vi "Package Class FG.vi"(8 "error in (no error)":errorcluster, 10 "Package Type (All)":string) -> (0 "error out":errorcluster, 2 "Package Class":refnum<class "PackageAbstract.lvclass">, 3 "Package Classes":T1(c390))   [LabVIEW 2020, in "GPack.lvlib"]
uses:
  GPack.lvlib
  PackageAbstract/PackageAbstract.lvclass
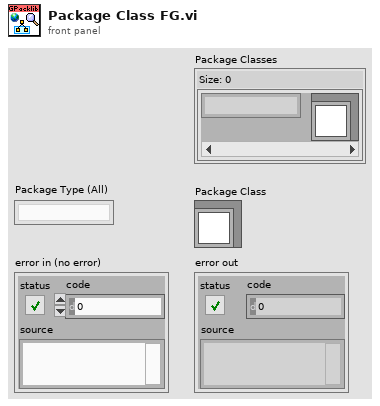
[diagram p1: front panel]
types:
  T1 = map{string, refnum<class "PackageAbstract.lvclass">}
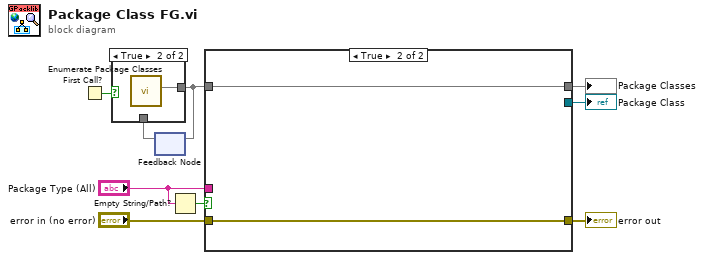
[diagram p0: block diagram]
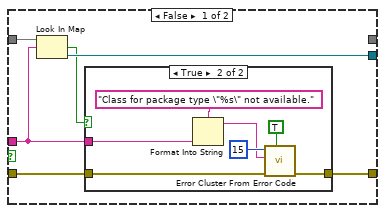
[diagram p3: hidden frame]
diagram:
  n1 = First Call?() -> (First Call?: T/F=w9:bool)
  n2 = feedback #1() -> (w8:T1)  [unwired: 1 in]
  n3 = case shown="True" w9 {
    tunnel: [w10 w11] -> w7
    tunnel: w8 -> [w10 _]
    frame False {
    }
    frame True {
      n4 = call "Enumerate Package Classes.vi"() -> ("Package Classes"=w11:T1)  [unwired: 11 in]
    }
  }
  n5 = feedback-in #1(w7) -> ()
  n6 = Empty String/Path?(string/path="Package Type (All)") -> (empty?=w3:bool)
  n7 = case shown="True" w3 {
    tunnel: w7 -> [w17 w26]
    tunnel: [w16 _] -> w6
    tunnel: "error in (no error)" -> [w14 w27]
    tunnel: [w13 w27] -> w4
    tunnel: "Package Type (All)" -> [w12 _]
    tunnel: [_ w26] -> w1
    frame False {
      n8 = Look In Map(map=w17, key=w12) -> (key not found?=w15:bool, value=w16:refnum<class "PackageAbstract.lvclass">)  [unwired: 1 in]
      n9 = case shown="True" w15 {
        tunnel: w14 -> [w18 w21]
        tunnel: [w18 w20] -> w13
        tunnel: w12 -> [_ w19]
        frame False {
        }
        frame True {
          n10 = Format Into String(format string="Class for package type \"%s\" not available.", w19) -> (resulting string=w22:string)  [unwired: 2 in, 1 out]
          n11 = call <vilib>:"Error Cluster From Error Code.vi"("show call chain? (False)"=TRUE, "error in (no error)"=w21, "error message (\"\")"=w22, "error code (0)"=15) -> ("error out"=w20:errorcluster)  [unwired: 5 in]
        }
      }
    }
    frame True {
    }
  }
  "error out" <- w4
  "Package Class" <- w6
  "Package Classes" <- w1
